vi "Build Responses Array.vi"(6 "RESTful VI configuration":T1={"Service VI Type"=enum."Web Method", "Load VI at statup"=TRUE, "Keep VI in memory"=TRUE, "Output type"=enum."Terminal", "Output format"=enum."XML", "Use headers"=TRUE, "Buffered"=TRUE, "eng_Load VI by name"=FALSE}, 8 "error in (no error)":errorcluster, 9 "VI Name":string, 10 "Controls and Indicators for XML":T6, 11 "Description in":T7) -> (0 "error out":errorcluster, 3 "Description out":T7)   [LabVIEW 2020, in "Web Service Description.lvlib"]
uses:
  <vilib>/AppBuilder/Engine/WebServiceDescription/Web Service Description.lvlib
  <vilib>/AppBuilder/Engine/WebServiceDescription/Web Service Description Info.ctl
  <vilib>/AppBuilder/Engine/WebServiceDescription/Response.ctl
  <vilib>/AppBuilder/AB_Classes/Source/RESTfulVI/Configure_RESTfulVI/AB_RESTful_OutputFormat.ctl
  <vilib>/AppBuilder/AB_Classes/Source/RESTfulVI/Configure_RESTfulVI/AB_RESTful_OutputType.ctl
  <vilib>/AppBuilder/Engine/WebServiceDescription/Terminal Info.ctl
  <vilib>/AppBuilder/Engine/WebServiceDescription/LVDataTypes/LVType/LVType.lvclass
  <vilib>/AppBuilder/Engine/WebServiceDescription/URL Mapping Info.ctl
  <vilib>/AppBuilder/AB_Classes/RESTful/AB_RESTful_HTTPMethodType.ctl
  <vilib>/AppBuilder/AB_Classes/Source/RESTfulVI/Configure_RESTfulVI/AB_RESTful_Configuration.ctl
  <vilib>/AppBuilder/AB_Classes/Source/RESTfulVI/Configure_RESTfulVI/AB_RESTful_VIType.ctl
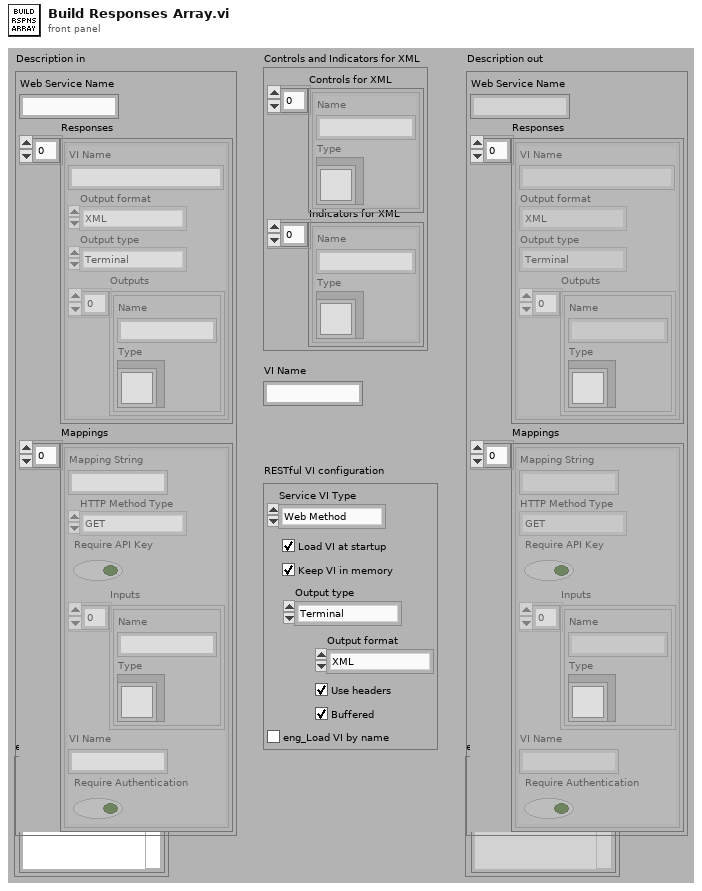
[diagram p1: front panel]
types:
  T1 = typedef "AB_RESTful_Configuration.ctl" = cluster{"Service VI Type":T2, "Load VI at statup":bool, "Keep VI in memory":bool, "Output type":T3, "Output format":T4, "Use headers":bool, "Buffered":bool, "eng_Load VI by name":bool}
  T2 = typedef "AB_RESTful_VIType.ctl" = enum32{"Web Method", "Auxiliary", "eng_Internal", "eng_Content"}
  T3 = typedef "AB_RESTful_OutputType.ctl" = enum32{"Terminal", "Stream"}
  T4 = typedef "AB_RESTful_OutputFormat.ctl" = enum32{"XML", "Text", "HTML", "JSON"}
  T5 = typedef "Web Service Description.lvlib/Terminal Info.ctl" = cluster{"Name":string, "Type":refnum<class "LVType.lvclass">}
  T6 = cluster{"Controls for XML":T5[], "Indicators for XML":T5[]}
  T7 = typedef "Web Service Description.lvlib/Web Service Description Info.ctl" = cluster{"Web Service Name":string, "Responses":T8[], "Mappings":T9[]}
  T8 = typedef "Web Service Description.lvlib/Response.ctl" = cluster{"VI Name":string, "Output format":T4, "Output type":T3, "Outputs":T5[]}
  T9 = typedef "Web Service Description.lvlib/URL Mapping Info.ctl" = cluster{"Mapping String":string, "HTTP Method Type":T10, "Require API Key":bool, "Inputs":T5[], "VI Name":string, "Require Authentication":bool}
  T10 = typedef "AB_RESTful_HTTPMethodType.ctl" = enum32{"GET", "POST", "PUT", "DELETE"}
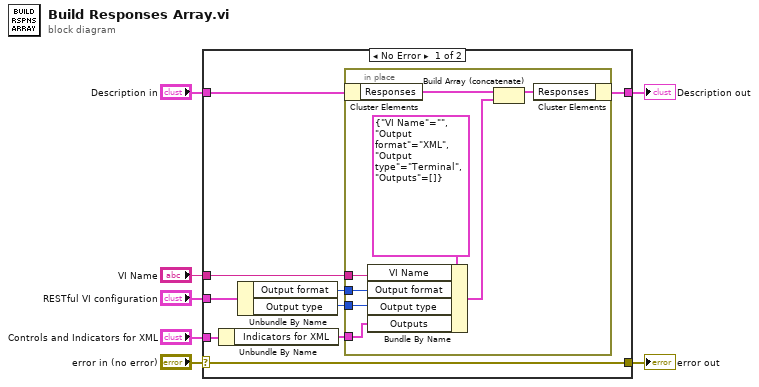
[diagram p0: block diagram]
diagram:
  n1 = case shown="No Error" "error in (no error)" {
    selector: "error in (no error)" -> [w8 w26]
    tunnel: [w8 w26] -> w6
    tunnel: "Description in" -> [w14 w25]
    tunnel: [w13 w25] -> w4
    tunnel: "Controls and Indicators for XML" -> [w16 _]
    tunnel: "RESTful VI configuration" -> [w12 _]
    tunnel: "VI Name" -> [w10 _]
    frame No Error {
      n2 = Unbundle By Name(w16) -> ("Indicators for XML"=w15:T5[])
      n3 = Unbundle By Name(w12) -> ("Output format"=w11:T4, "Output type"=w9:T3)
      n4 = in-place {
        in-place-border: w15 -> [w23]
        in-place-border: w11 -> [w19]
        in-place-border: w10 -> [w18]
        in-place-border: w9 -> [w17]
        n5 = in-place-cluster #1(w14) -> ("Responses"=w22:T8[])
        n6 = Bundle By Name(cluster=T8 {"VI Name"="", "Output format"=enum."XML", "Output type"=enum."Terminal", "Outputs"=[]} ("Response"), "VI Name"=w18, "Output format"=w19, "Output type"=w17, "Outputs"=w23) -> (w20:T8)
        n7 = Build Array (concatenate)(w22, w20) -> (w21:T8[])
        n8 = in-place-cluster #1("Responses"=w21) -> (w13:T7)
      }
    }
    frame Error {
    }
  }
  "error out" <- w6
  "Description out" <- w4
